vi "Init Msg.vi"(10 "Msg Input":refnum<class "Msg Input.lvclass">) -> (3 "TEMPLATE Msg out":refnum<class "TEMPLATE Msg.lvclass">)   [LabVIEW 2025, in "_Template.lvlib" / "Templates.lvlib" / "TEMPLATE Msg.lvlib" / "TEMPLATE Msg.lvlib" / "TEMPLATE Msg.lvclass"]
uses:
  TEMPLATE Msg.lvclass
  jettl/jettl/Msg Input/Msg Input.lvclass
  TEMPLATE Msg.lvclass/TEMPLATE Msg.ctl
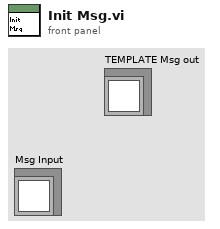
[diagram p1: front panel]
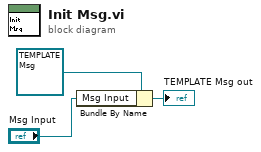
[diagram p0: block diagram]
diagram:
  n1 = Bundle By Name(cluster=refnum<class "TEMPLATE Msg.lvclass"> refnum ("TEMPLATE Msg out"), "Msg Input"="Msg Input") -> (→"TEMPLATE Msg out":refnum<class "TEMPLATE Msg.lvclass">)
